vi "Implementing_FFT.vi"() -> ()   [LabVIEW 2016]
uses:
  <vilib>/Analysis/NI_AALBase.lvlib
  <vilib>/Analysis/NI_AALPro.lvlib
  <vilib>/Analysis/2dsp.llb/Decimate (single shot, DBL).vi
  <vilib>/Analysis/3filter.llb/Butterworth Filter (DBL).vi
  <vilib>/Analysis/2dsp.llb/Real FFT.vi
  <vilib>/Utility/file.llb/Read Delimited Spreadsheet (DBL).vi
panel:
  in  "Resample factor":i32=2
  in  "Amplitude":dbl=0.3
  in  "Resample?":bool
  in  "Apply filter?":bool
  in  "Add sine wave noise?":bool
  in  "Add white noise?":bool
  out "Time Domain Signal":cluster{i32, dbl, dbl[]}(graph)={0, 0.008, []}
  in  "Sine wave\nfrequency":dbl=60.0
  in  "Cutoff\n Frequency":dbl=20.0
  in  "Amplitude":dbl=0.01
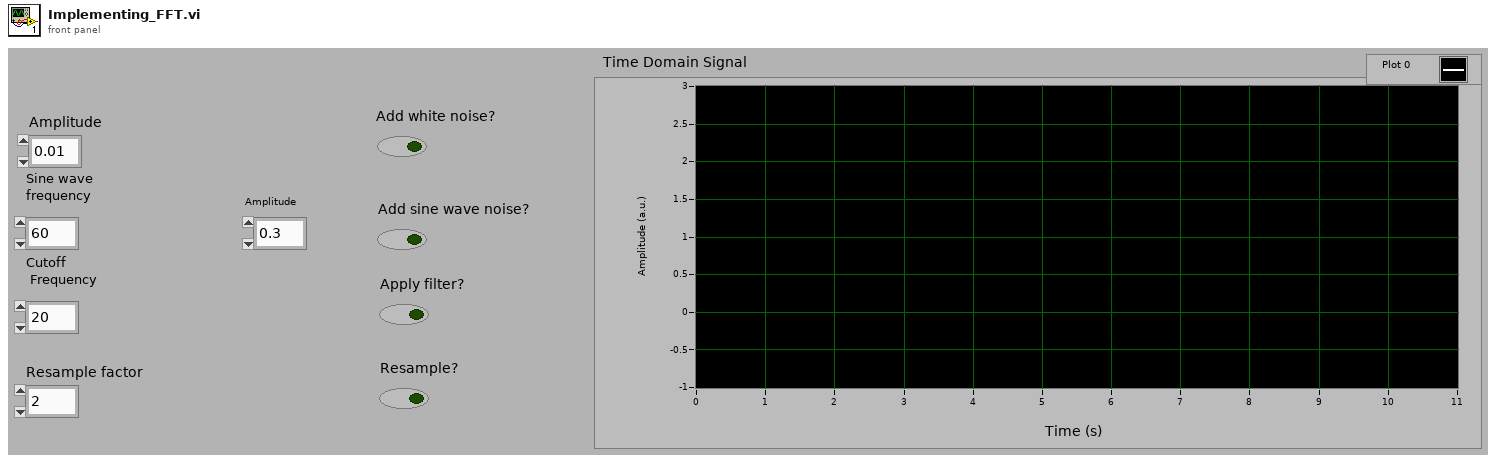
[diagram p1: front panel]
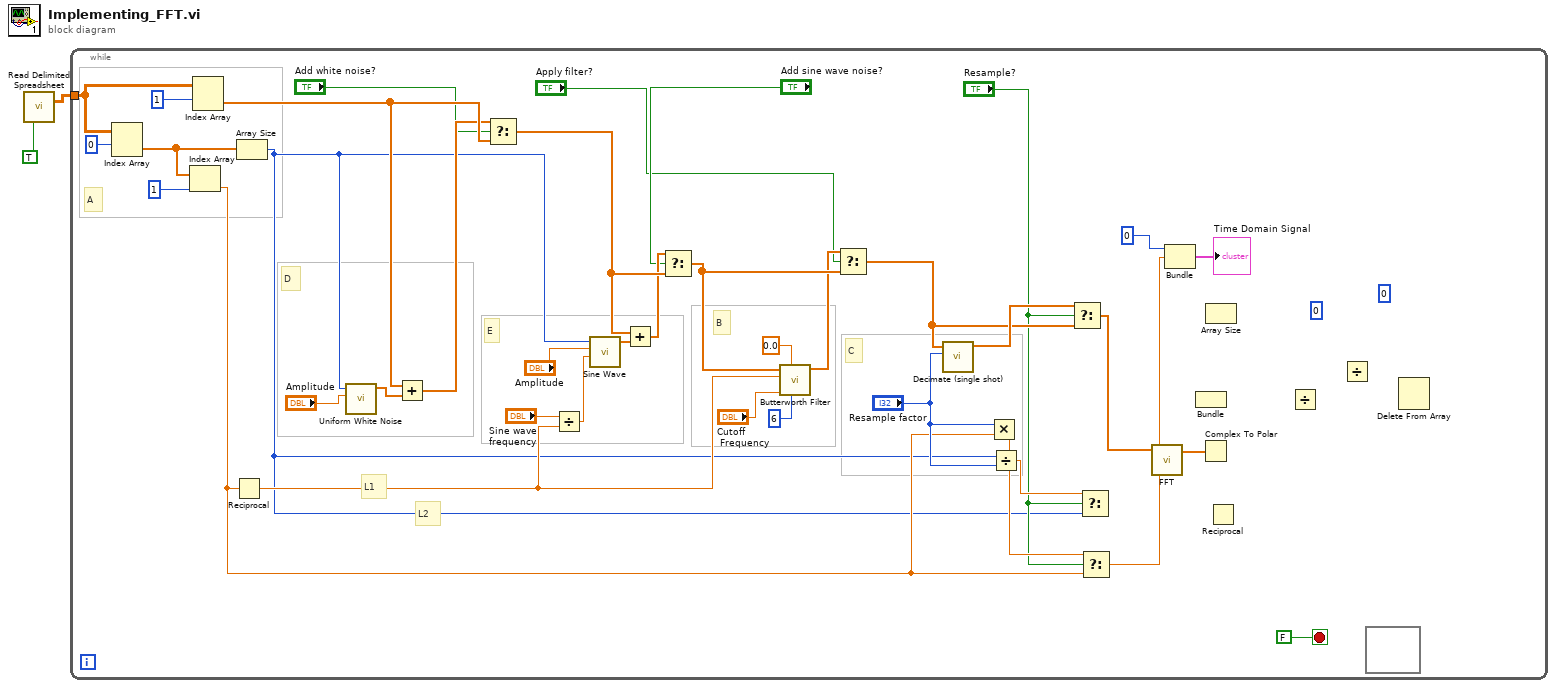
[diagram p0: block diagram]
diagram:
  n1 = call-poly <vilib>:"Read Delimited Spreadsheet.vi"("transpose? (F)"=TRUE ("Boolean")) -> ("all rows"=w1:dbl[][])  [unwired: 9 in, 5 out]
  n2 = while {
    tunnel: w1 -> [w20]
    stop <- FALSE stop-if-true
    (unwired) 0
    (unwired) 0
    # "L2"
    # "L1"
    # "C"
    # "B"
    # "E"
    # "D"
    # "A"
    n3 = Index Array(array=w20, index (row)=0) -> (element=w16:dbl[])  [unwired: 1 in]
    n4 = Index Array(array=w16, index=1) -> (element=w10:dbl)
    n5 = Index Array(array=w20, index (row)=1) -> (element=w32:dbl[])  [unwired: 1 in]
    n6 = Reciprocal(x=w10) -> (1/x=w17:dbl)
    n7 = Array Size(array=w16) -> (size(s)=w5:i32)
    n8 = call <vilib>:"Uniform White Noise.vi"("amplitude"="Amplitude", "samples"=w5) -> ("uniform white noise"=w3:dbl[])  [unwired: 8 in, 1 out]
    n9 = Add(x=w32, y=w3) -> (x+y=w31:dbl[])
    n10 = Select(t=w31, s="Add white noise?", f=w32) -> (s? t:f=w29:dbl[])
    n11 = Divide(x="Sine wave\nfrequency", y=w17) -> (x/y=w36:dbl)
    n12 = call <vilib>:"Sine Wave.vi"("samples"=w5, "amplitude"="Amplitude", "frequency"=w36) -> ("sine wave"=w34:dbl[])  [unwired: 2 in, 2 out]
    n13 = Add(x=w29, y=w34) -> (x+y=w28:dbl[])
    n14 = Select(t=w28, s="Add sine wave noise?", f=w29) -> (s? t:f=w26:dbl[])
    n15 = call-poly <vilib>:"Butterworth Filter.vi"("order"=6 ("Filter order"), "filter type"=0.0 ("Filter Type"), "low cutoff freq: fl"="Cutoff\n Frequency", "sampling freq: fs"=w17, "X"=w26) -> ("Filtered X"=w25:dbl[])  [unwired: 2 in, 2 out]
    n16 = Select(t=w25, s="Apply filter?", f=w26) -> (s? t:f=w22:dbl[])
    n17 = call-poly <vilib>:"Decimate (single shot).vi"("decimating factor"="Resample factor", "X"=w22) -> ("Decimated Array"=w23:dbl[])  [unwired: 1 in, 8 out]
    n18 = Multiply(x="Resample factor", y=w10) -> (x*y=w14:dbl)
    n19 = Divide(x=w5, y="Resample factor") -> (x/y=w12:dbl)
    n20 = Select(t=w23, s="Resample?", f=w22) -> (s? t:f=w7:dbl[])
    n21 = Select(t=w12, s="Resample?", f=w5) -> ()  [unwired: 1 out]
    n22 = Select(t=w14, s="Resample?", f=w10) -> (s? t:f=w8:dbl)
    n23 = call-poly <vilib>:"FFT.vi"("X"=w7) -> ("FFT {X}"=w6:cdb[])  [unwired: 9 in, 1 out]
    n24 = Bundle(0, "Numeric"=w8) -> (→"Time Domain Signal":cluster{i32, "Numeric":dbl, void})  [unwired: 2 out]
    n25 = Bundle() -> ()  [unwired: 3 in, 1 out]
    n26 = Complex To Polar(r * e^(i*theta)=w6) -> ()  [unwired: 2 out]
    n27 = Array Size() -> ()  [unwired: 1 in, 1 out]
    n28 = Reciprocal() -> ()  [unwired: 1 in, 1 out]
    n29 = Divide() -> ()  [unwired: 2 in, 1 out]
    n30 = Divide() -> ()  [unwired: 2 in, 1 out]
    n31 = formula code=""() -> ()
    n32 = Delete From Array() -> ()  [unwired: 3 in, 2 out]
  }
